vi "ALTS-2015 DB Part Details Driver.vi"(7 "Operation":T1=enum."Read DB", 8 "error in (no error)":errorcluster, 11 "Serial Number":string) -> (0 "error out":errorcluster, 1 "Adapter Plate Size":i32, 2 "Air Leak Test Type":i32, 3 "S No Valid?":bool, 4 "Displacement Size":i32, 5 "Flange Size":i32)   [LabVIEW 2013]
doc: "Copyright © 2005, Soliton Technologies.\nAll rights reserved."
uses:
  Controls/ALTS-2015 DB Driver Options.ctl
  <vilib>/addons/database/Auxilliary.llb/DB Tools Parameter Info.ctl
  <vilib>/addons/database/Auxilliary.llb/DB Tools DataTypes.ctl
  <vilib>/addons/database/Auxilliary.llb/DB Tools Parameter Dir.ctl
  Controls/ALTS-2015 LV2GBL Options.ctl
  <vilib>/addons/database/Command.llb/Cmd ObjectReference.ctl
  <vilib>/addons/database/Connection.llb/DB Tools Open Connec (Path).vi
  <vilib>/addons/database/Command.llb/Cmd Set Parameter Value (C).vi
  <vilib>/addons/database/Command.llb/Cmd Execute.vi
  <vilib>/addons/database/Recordset.llb/Rec Fetch Recordset Data (R).vi
  <vilib>/addons/database/Recordset.llb/Rec Destroy - Connection.vi
  <vilib>/Utility/file.llb/Read From Spreadsheet File (string).vi
  <vilib>/addons/database/Command.llb/Cmd Delete.vi
  <vilib>/addons/database/_DB Variant To Data/Database Variant To Data.xnode
  <vilib>/addons/database/NI_Database_API.lvlib
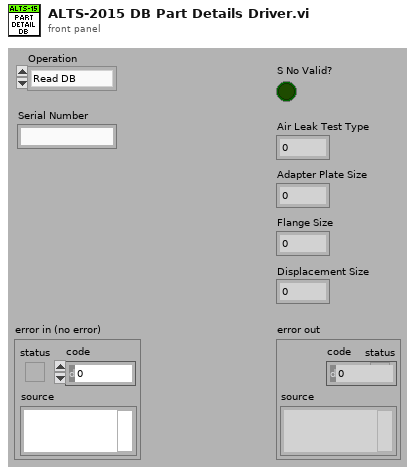
[diagram p1: front panel]
types:
  T1 = typedef "ALTS-2015 DB Driver Options.ctl" = enum16{"Init", "Read DB", "Close"}
  T2 = typedef "ALTS-2015 LV2GBL Options.ctl" = enum16{"Read all", "Write all"}
  T3 = typedef "NI_Database_API.lvlib/DB Tools Parameter Info.ctl" = cluster{"parameter name":string, "type":T4, "direction":T5, "value":variant}
  T4 = typedef "NI_Database_API.lvlib/DB Tools DataTypes.ctl" = enum16{"String", "Long (I32)", "Single (SGL)", "Double (DBL)", "Date/Time", "Binary"}
  T5 = typedef "NI_Database_API.lvlib/DB Tools Parameter Dir.ctl" = enum32{"Input", "Output", "Input/Output", "Return Value"}
  T6 = typedef "ALTS-2015 INI Configuration Cluster.ctl" = cluster{"Application":cluster{"Rerun Count":i32, "Workorder No":i32}, "Station Details":cluster{"Sensor Name 1":string, "Sensor Name 2":string, "Sensor Name 3":string, "Sensor Name 4":string, "Station1 Enable":bool, "Station2 Enable":bool, "Station3 Enable":bool, "Station4 Enable":bool}, "Database":cluster{"Database Connection Link":path, "Result Procedure":string, "User":string, "Password":string, "Prompt":bool, "Station 1 LT Result DB DSN Path":path, "Station 2 LT Result DB DSN Path":path, "Station 3 LT Result DB DSN Path":path, "Station 4 LT Result DB DSN Path":path, "AirLeakTestResult Procedure":string, "Serial Details Procedure":string}, "Simulation":cluster{"Simulate DAQ Hardware":bool, "Simulate Result DB Write":bool, "Simulate Scanner":bool, "Simulate OPC":bool, "Simulate LeakTek DB":bool, "Simulate Serial Details DB":bool, "Simulate Scanner DB Path":path, "Simulate AirLeakLookup DB Path":path}, "Barcode Scanner1":cluster{"Scanner IP":string, "Scanner Port":u16, "#Bytes to Read":i32}, "Barcode Scanner2":cluster{"Enabled?":bool, "Scanner IP":string, "Scanner Port":u16, "#Bytes to Read":i32}}
  T7 = typedef "NI_Database_API.lvlib/Conn ObjectReference.ctl" = refnum<k1>
  T8 = typedef "NI_Database_API.lvlib/Cmd ObjectReference.ctl" = refnum<k1>
  T9 = typedef "NI_Database_API.lvlib/Cmd-Rec Object Reference.ctl" = refnum<k1>
  T10 = typedef "NI_Database_API.lvlib/Cmd-Rec Data Members.ctl" = cluster{"recordset reference":T11, "command reference":T8}
  T11 = typedef "NI_Database_API.lvlib/Rec ObjectReference.ctl" = refnum<k1>
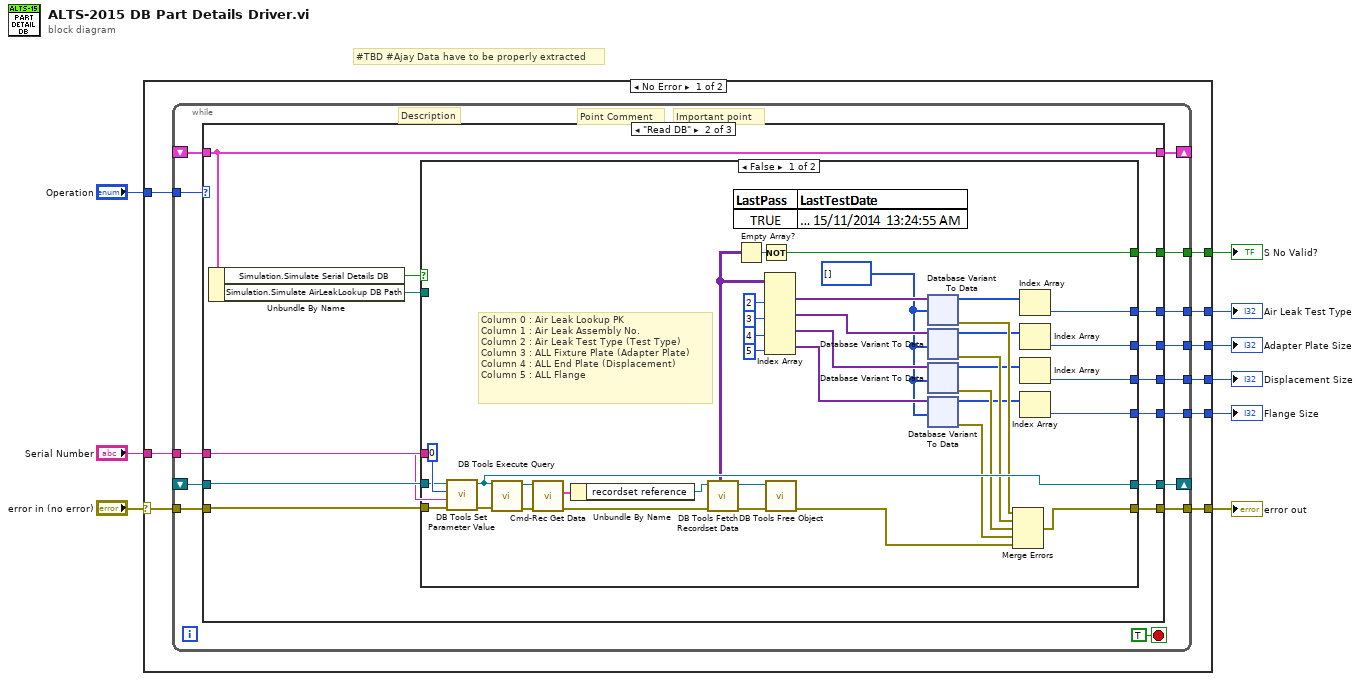
[diagram p0: block diagram]
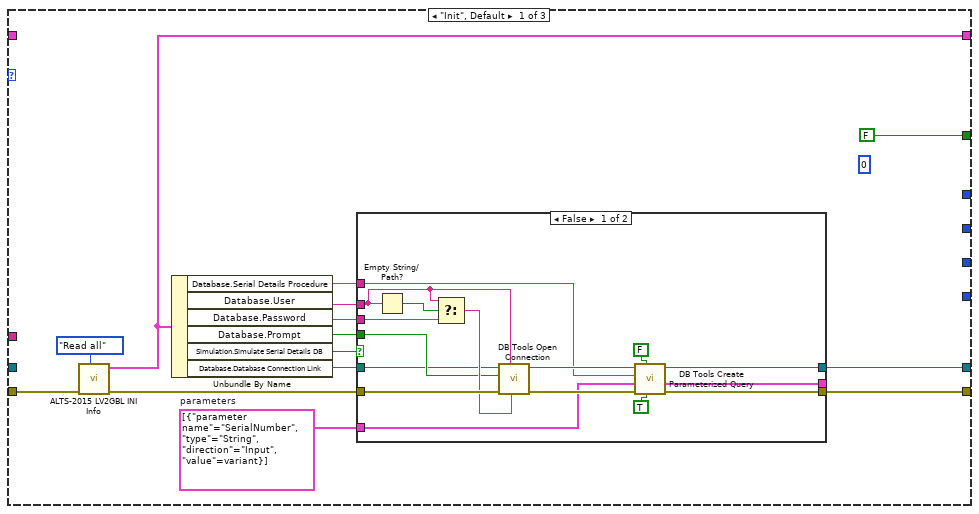
[diagram p2: hidden frame]
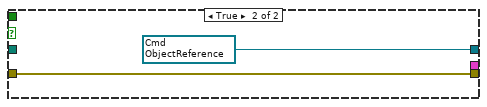
[diagram p3: hidden frame]
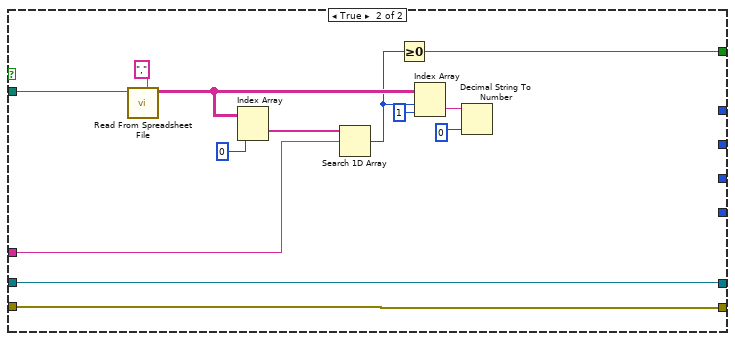
[diagram p4: hidden frame]
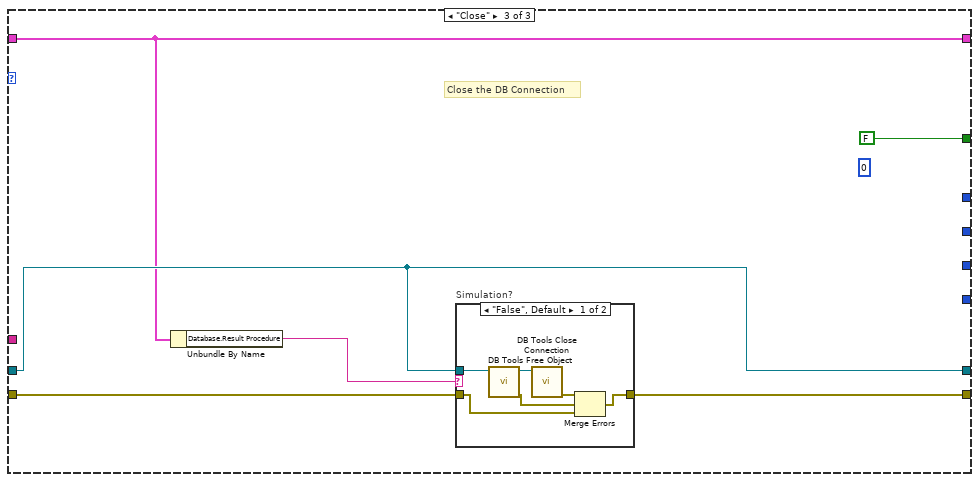
[diagram p5: hidden frame]
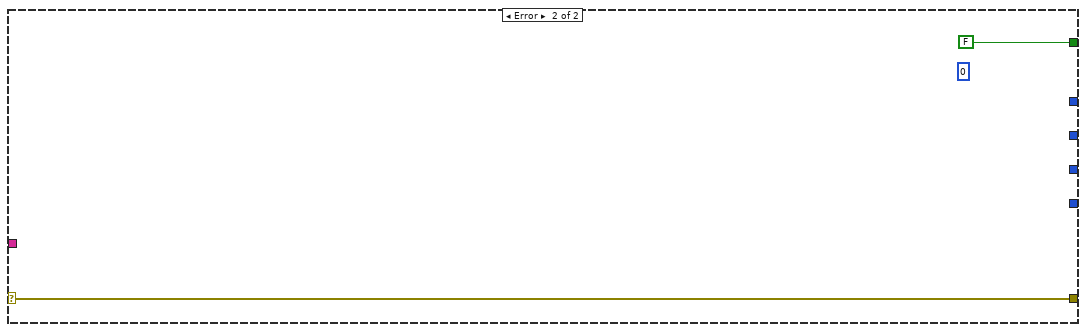
[diagram p7: hidden frame]
diagram:
  # "#TBD #Ajay Data have to be properly extracted"
  n1 = case shown="No Error" "error in (no error)" {
    selector: "error in (no error)" -> [w17 w296]
    tunnel: [w18 w296] -> w8
    tunnel: "Operation" -> [w16 _]
    tunnel: "Serial Number" -> [w15 _]
    tunnel: [w14 FALSE] -> w5
    tunnel: [w13 _] -> w1
    tunnel: [w12 _] -> w2
    tunnel: [w11 _] -> w4
    tunnel: [w10 _] -> w3
    frame No Error {
      # "Point Comment"
      # "Important point"
      # "Description"
      n2 = while {
        tunnel: [w31] -> w18
        shift-right: [w30] -> _
        shift-left: _ -> [w29]
        tunnel: w17 -> [w28]
        tunnel: w16 -> [w27]
        tunnel: w15 -> [w26]
        tunnel: [w25] -> w14
        shift-right: [w24] -> _
        shift-left: _ -> [w23]
        tunnel: [w22] -> w13
        tunnel: [w21] -> w12
        tunnel: [w20] -> w11
        tunnel: [w19] -> w10
        stop <- TRUE stop-if-true
        n3 = case shown="\"Read DB\"" w27 {
          tunnel: w28 -> [w37 w76 w283]
          tunnel: [w46 w77 w287] -> w31
          tunnel: [w45 w74 w286] -> w30
          tunnel: w29 -> [_ w75 w286]
          tunnel: w26 -> [_ w73 _]
          tunnel: [FALSE w70 FALSE] -> w25
          tunnel: [w34 w69 w282] -> w24
          tunnel: w23 -> [_ w69 w282]
          tunnel: [_ w68 _] -> w22
          tunnel: [_ w67 _] -> w21
          tunnel: [_ w66 _] -> w20
          tunnel: [_ w65 _] -> w19
          frame "Init", Default {
            (unwired) u16 0 ("data")
            w38 = T3[] [{"parameter name"="SerialNumber", "type"=enum."String", "direction"=enum."Input", "value"=variant}]  # parameters
            n4 = call "ALTS-2015 LV2GBL INI Info.vi"("Options"=ALTS-2015_LV2GBL_Options."Read all", "error in"=w37) -> ("error out"=w36:errorcluster, "Configuration Cluster Out"=w34:T6)  [unwired: 8 in]
            n5 = Unbundle By Name(w34) -> ("Database.Serial Details Procedure"=w39:string, "Database.User"=w42:string, "Database.Password"=w41:string, "Database.Prompt"=w40:bool, "Simulation.Simulate Serial Details DB"=w43:bool, "Database.Database Connection Link"=w44:path)
            n6 = case shown="False" w43 {
              tunnel: [w51 w64] -> w46
              tunnel: [w52 w63] -> w45
              tunnel: w44 -> [w47 _]
              tunnel: w36 -> [w62 w64]
              tunnel: w42 -> [w59 _]
              tunnel: w41 -> [w58 _]
              tunnel: w40 -> [w57 _]
              tunnel: w39 -> [w54 _]
              tunnel: w38 -> [w48 _]
              tunnel: [w49 _] -> _
              frame False {
                n7 = Empty String/Path?(string/path=w59) -> (empty?=w61:bool)
                n8 = Select(t=w59, s=w61, f=w58) -> (s? t:f=w60:string)
                n9 = call-poly <vilib>:"DB Tools Open Connection.vi"("password"=w60, "userID"=w59, "error in (no error)"=w62, "prompt? (F)"=w57, "connection information"=w47) -> ("error out"=w50:errorcluster, "connection reference"=w55:T7)  [unwired: 3 in]
                n10 = call <vilib>:"DB Tools Create Parameterized Query.vi"("stored procedure? (F)"=TRUE ("stored procedure? (f)"), "auto-detect parameters? (F)"=FALSE ("auto-detect parameters? (f)"), "error in (no error)"=w50, "parameters"=w48, "SQL query"=w54, "connection reference"=w55) -> ("error out"=w51:errorcluster, "parameters out"=w49:T3[], "command reference"=w52:T8)  [unwired: 1 in]
              }
              frame True {
                w63 = T8 refnum items=["Command"] ("command reference")
              }
            }
          }
          frame "Read DB" {
            n11 = Unbundle By Name(w69) -> ("Simulation.Simulate Serial Details DB"=w72:bool, "Simulation.Simulate AirLeakLookup DB Path"=w71:path)
            n12 = case shown="False" w72 {
              tunnel: [w108 w281] -> w77
              tunnel: w76 -> [w110 w281]
              tunnel: w75 -> [w111 w280]
              tunnel: [w101 w280] -> w74
              tunnel: w73 -> [w114 w275]
              tunnel: w71 -> [_ w279]
              tunnel: [w100 w270] -> w70
              tunnel: [w83 _] -> w68
              tunnel: [w84 _] -> w67
              tunnel: [w79 _] -> w66
              tunnel: [w78 _] -> w65
              frame False {
                w82 = i32[] []
                # "Column 0 : Air Leak Lookup PK\nColumn 1 : Air Leak Assembly No.\nColumn 2 : Air Leak Test Type (Test Type)\nColumn 3 : ALL Fixture Plate (Adapter Plate)\nColumn 4 : ALL End Plate (Displacement)\nColumn 5 : ALL Flange"
                n13 = call-poly <vilib>:"DB Tools Set Parameter Value.vi"("error in (no error)"=w110, "value"=w114, "parameter index"=0, "command reference"=w111) -> ("error out"=w109:errorcluster, "command reference out"=w101:T8)  [unwired: 4 in]
                n14 = call-poly <vilib>:"DB Tools Execute Query.vi"("error in (no error)"=w109, "command reference"=w101) -> ("error out"=w103:errorcluster, "command-recordset reference"=w104:T9)  [unwired: 6 in]
                n15 = call <vilib>:"Cmd-Rec Get Data.vi"("error in (no error)"=w103, "command-recordset reference"=w104) -> ("error out"=w102:errorcluster, "data"=w106:T10)  [unwired: 2 in, 2 out]
                n16 = Unbundle By Name(w106) -> ("recordset reference"=w105:T11)
                n17 = call-poly <vilib>:"DB Tools Fetch Recordset Data.vi"("error in (no error)"=w102, "recordset reference"=w105) -> ("error out"=w112:errorcluster, "recordset data"=w99:variant[][], "recordset reference out"=w115:T11)  [unwired: 3 in]
                n18 = Empty Array?(array=w99) -> (empty?=w113:bool)
                n19 = Not(x=w113) -> (.not. x?=w100:bool)
                n20 = Index Array(array=w99, index (col) #1=2 ("disabled index (col)"), index (col) #2=3 ("disabled index (col)"), index (col) #3=4 ("disabled index (col)"), index (col) #4=5 ("disabled index (col)")) -> (element #1=w94:variant[], element #2=w93:variant[], element #3=w92:variant[], element #4=w91:variant[])  [unwired: 4 in]
                n21 = call-poly <vilib>:"DB Tools Free Object.vi"("error in (no error)"=w112, "recordset reference"=w115) -> ("error out"=w107:errorcluster)  [unwired: 8 in, 1 out]
                n22 = xnode "Database Variant To Data"("database variant"=w94, "type"=w82) -> ("data"=w81:i32[], "error out"=w90:errorcluster)  [unwired: 1 in]
                n23 = xnode "Database Variant To Data"("database variant"=w93, "type"=w82) -> ("data"=w80:i32[], "error out"=w89:errorcluster)  [unwired: 1 in]
                n24 = xnode "Database Variant To Data"("database variant"=w92, "type"=w82) -> ("data"=w85:i32[], "error out"=w88:errorcluster)  [unwired: 1 in]
                n25 = xnode "Database Variant To Data"("database variant"=w91, "type"=w82) -> ("data"=w86:i32[], "error out"=w87:errorcluster)  [unwired: 1 in]
                n26 = Merge Errors(w90, w89, w88, w87, w107) -> (w108:errorcluster)
                n27 = Index Array(array=w81) -> (element=w79:i32)  [unwired: 1 in]
                n28 = Index Array(array=w80) -> (element=w78:i32)  [unwired: 1 in]
                n29 = Index Array(array=w85) -> (element=w84:i32)  [unwired: 1 in]
                n30 = Index Array(array=w86) -> (element=w83:i32)  [unwired: 1 in]
              }
              frame True {
                n31 = call-poly <vilib>:"Read From Spreadsheet File.vi"("delimiter (\\t)"="," ("delimiter (\\t)"), "file path (dialog if empty)"=w279) -> ("all rows"=w274:string[][])  [unwired: 5 in, 4 out]
                n32 = Index Array(array=w274, index (col)=0 ("disabled index (col)")) -> (element=w276:string[])  [unwired: 1 in]
                n33 = Search 1D Array(1D array=w276, element=w275) -> (index of element=w271:i32)  [unwired: 1 in]
                n34 = Greater Or Equal To 0?(x=w271) -> (x >= 0?=w270:bool)
                n35 = Index Array(array=w274, index (row)=w271, index (col)=1 ("disabled index (col)")) -> (element=w272:string)
                n36 = Decimal String To Number(string=w272, default (0L)=u16 0 ("number")) -> ()  [unwired: 1 in, 2 out]
              }
            }
          }
          frame "Close" {
            (unwired) u16 0 ("data")
            # "Close the DB Connection"
            n37 = Unbundle By Name(w282) -> ("Database.Result Procedure"=w285:string)
            n38 = case "Simulation?" shown="\"False\", Default" w285 {
              tunnel: [w288 w294] -> w287
              tunnel: w286 -> [w293 _]
              tunnel: w283 -> [w289 w294]
              frame "False", Default {
                n39 = call-poly <vilib>:"DB Tools Free Object.vi"("command reference"=w293) -> ("error out"=w290:errorcluster, "connection reference"=w292:T7)  [unwired: 9 in]
                n40 = call <vilib>:"DB Tools Close Connection.vi"("connection reference"=w292) -> ("error out"=w291:errorcluster)  [unwired: 6 in]
                n41 = Merge Errors(w291, w290, w289) -> (w288:errorcluster)
              }
              frame "True" {
              }
            }
          }
        }
      }
    }
    frame Error {
      (unwired) u16 0 ("data")
    }
  }
  "error out" <- w8
  "S No Valid?" <- w5
  "Adapter Plate Size" <- w3
  "Air Leak Test Type" <- w4
  "Flange Size" <- w1
  "Displacement Size" <- w2
